vi "Generate DCIR Plots.vi"(8 "error in (no error)":errorcluster, 10 "DCIR Parameters":T1={"Initial SoC (%)"=650.0, "Pulse Mode"=2, "Pulse Current (A)"=1000.0, "Pulse Duration (S)"=500.0} {"Pulse Mode" items=["Discharge"=1, "Charge"=2]; "Initial SoC (%)" min=0.0 max=100.0}, 11 "TDMS Data File":path) -> (0 "error out":errorcluster, 3 "DCIR Nyquist":cluster{dbl[], dbl[]}(graph))   [LabVIEW 2023, in "DCIR_HPPC.lvclass"]
uses:
  HPPC Parameters.ctl
  HPPC Mode.ctl
  <vilib>/Analysis/baseanly.llb/Mean (DBL).vi
  <vilib>/Analysis/2dsp.llb/Real FFT.vi
  DCIR_HPPC.lvclass
  DCIR_HPPC.lvclass/DCIR_HPPC.ctl
  <vilib>/Analysis/NI_AALBase.lvlib
  <vilib>/Analysis/NI_AALPro.lvlib
panel:
  out "dF":dbl
  out "frequency (hz)":dbl
  out "period (seconds)":dbl format="%#_6f"
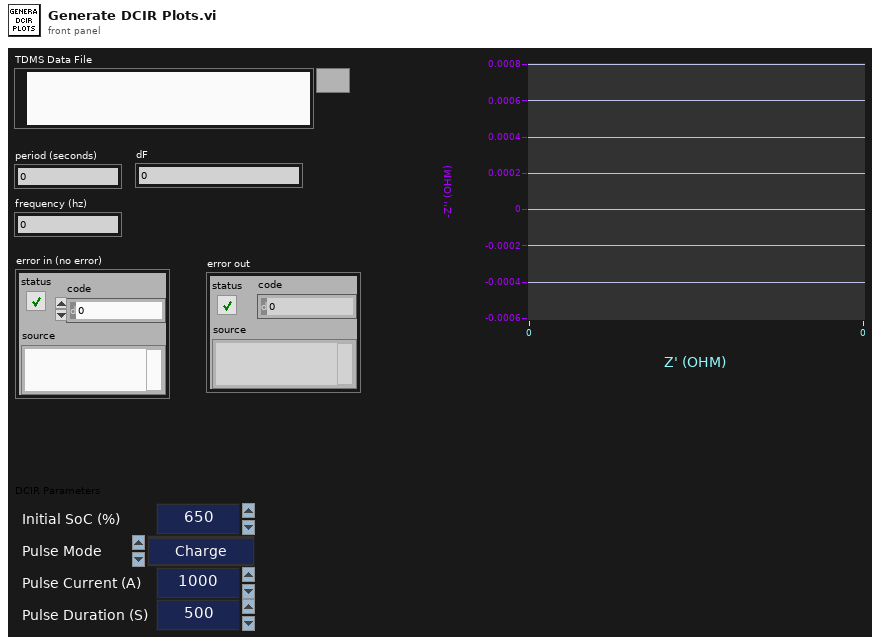
[diagram p1: front panel]
types:
  T1 = typedef "DCIR_HPPC.lvclass/HPPC Parameters.ctl" = cluster{"Initial SoC (%)":dbl, "Pulse Mode":T2, "Pulse Current (A)":dbl, "Pulse Duration (S)":dbl}
  T2 = typedef "DCIR_HPPC.lvclass/HPPC Mode.ctl" = u16
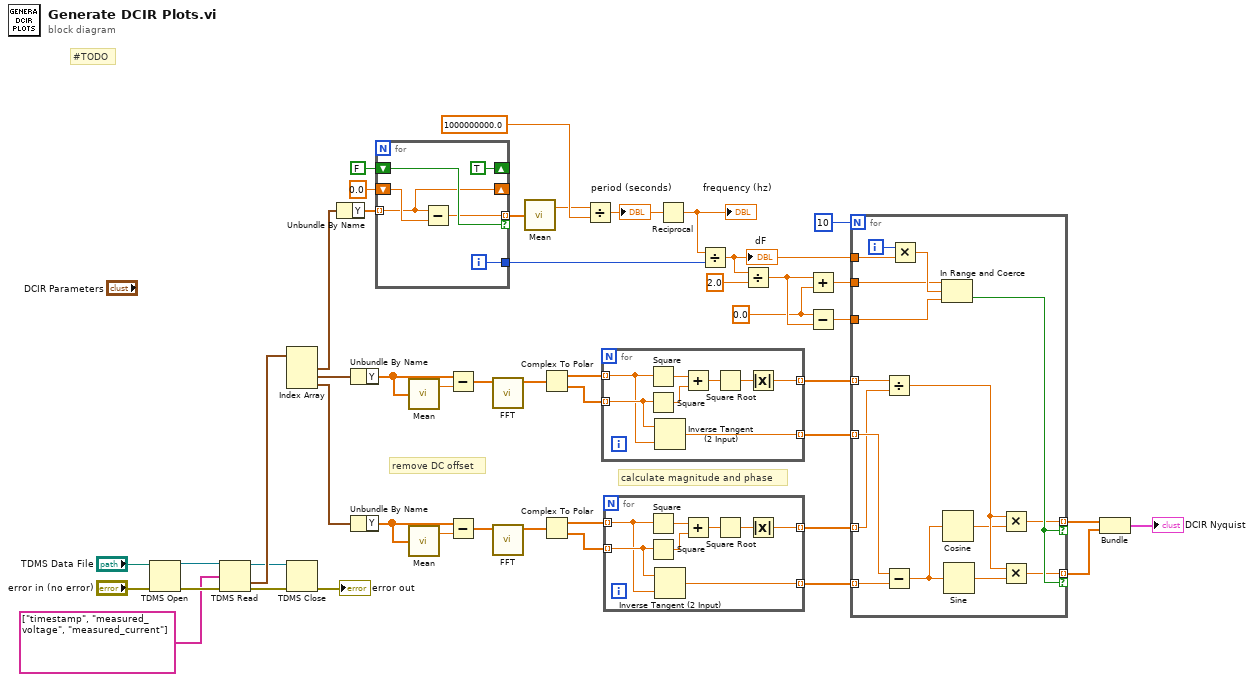
[diagram p0: block diagram]
diagram:
  w2 = 0.0 ("x")
  # "#TODO"
  # "calculate magnitude and phase"
  # "remove DC offset"
  n1 = TDMS Open(8:"error in (no error)", 11:"TDMS Data File") -> (0:w45:errorcluster, 3:w44:refnum<k34>)  [unwired: 5 in]
  n2 = TDMS Read(0:w44, 7:string[] ["timestamp", "measured_voltage", "measured_current"] ("channel name(s) in"), 11:w45) -> (4:w26:refnum<k34>, 10:w42:waveform(dbl)[], 15:w27:errorcluster)  [unwired: 5 in, 3 out]
  n3 = Index Array(array=w42) -> (element #1=w41:waveform(dbl), element #2=w32:waveform(dbl), element #3=w34:waveform(dbl))  [unwired: 3 in]
  n4 = TDMS Close(8:w27, 11:w26) -> (0:→"error out":errorcluster)  [unwired: 1 out]
  n5 = Unbundle By Name(w41) -> ("Y"=w40:dbl[])
  n6 = Unbundle By Name(w32) -> ("Y"=w22:dbl[])
  n7 = Unbundle By Name(w34) -> ("Y"=w18:dbl[])
  n8 = for {
    tunnel: w40 -> [w50] mode=indexing
    tunnel: [w49] -> w38 mode=indexing if=w52
    shift-right: [w50] -> _
    shift-left: 0.0 -> [w51]
    shift-right: [TRUE] -> _
    shift-left: FALSE -> [w52]
    tunnel: [w48] -> w14
    i -> [w48]
    n9 = Subtract(x=w50, y=w51) -> (x-y=w49:dbl)
  }
  n10 = call-poly <vilib>:"Mean.vi"("X"=w22) -> ("mean"=w21:dbl)  [unwired: 1 out]
  n11 = call-poly <vilib>:"Mean.vi"("X"=w18) -> ("mean"=w19:dbl)  [unwired: 1 out]
  n12 = Subtract(x=w22, y=w21) -> (x-y=w20:dbl[])
  n13 = Subtract(x=w18, y=w19) -> (x-y=w17:dbl[])
  n14 = call-poly <vilib>:"FFT.vi"("X"=w20) -> ("FFT {X}"=w13:cdb[])  [unwired: 9 in, 1 out]
  n15 = call-poly <vilib>:"FFT.vi"("X"=w17) -> ("FFT {X}"=w33:cdb[])  [unwired: 9 in, 1 out]
  n16 = call-poly <vilib>:"Mean.vi"("X"=w38) -> ("mean"=w37:dbl)  [unwired: 1 out]
  n17 = Complex To Polar(r * e^(i*theta)=w13) -> (r=w12:dbl[], theta=w28:dbl[])
  n18 = Complex To Polar(r * e^(i*theta)=w33) -> (r=w11:dbl[], theta=w31:dbl[])
  n19 = Divide(x=w37, y=1000000000.0) -> (x/y=w30:dbl)
  "period (seconds)" <- w30
  n20 = for {
    tunnel: w12 -> [w55] mode=indexing
    tunnel: w28 -> [w56] mode=indexing
    tunnel: [w57] -> w16 mode=indexing
    tunnel: [w54] -> w24 mode=indexing
    n21 = Square(x=w55) -> (x^2=w61:dbl)
    n22 = Square(x=w56) -> (x^2=w60:dbl)
    n23 = Inverse Tangent (2 Input)(1:w55, 2:w56) -> (0:w54:dbl)
    n24 = Add(x=w61, y=w60) -> (x+y=w59:dbl)
    n25 = Square Root(x=w59) -> (sqrt(x)=w58:dbl)
    n26 = Absolute Value(x=w58) -> (abs(x)=w57:dbl)
  }
  n27 = for {
    tunnel: w11 -> [w63] mode=indexing
    tunnel: w31 -> [w64] mode=indexing
    tunnel: [w65] -> w29 mode=indexing
    tunnel: [w62] -> w23 mode=indexing
    n28 = Square(x=w63) -> (x^2=w69:dbl)
    n29 = Square(x=w64) -> (x^2=w68:dbl)
    n30 = Inverse Tangent (2 Input)(1:w63, 2:w64) -> (0:w62:dbl)
    n31 = Add(x=w69, y=w68) -> (x+y=w67:dbl)
    n32 = Square Root(x=w67) -> (sqrt(x)=w66:dbl)
    n33 = Absolute Value(x=w66) -> (abs(x)=w65:dbl)
  }
  n34 = Reciprocal(x=w30) -> (1/x=w15:dbl)
  "frequency (hz)" <- w15
  n35 = Divide(x=w15, y=w14) -> (x/y=w10:dbl)
  "dF" <- w10
  n36 = Divide(x=w10, y=2.0) -> (x/y=w8:dbl)
  n37 = Add(x=w8, y=w2) -> (x+y=w6:dbl)
  n38 = Subtract(x=w2, y=w8) -> (x-y=w7:dbl)
  n39 = for {
    N: 10 -> [_]
    tunnel: w16 -> [w80] mode=indexing
    tunnel: w29 -> [w78] mode=indexing
    tunnel: w24 -> [w79] mode=indexing
    tunnel: w23 -> [w81] mode=indexing
    tunnel: [w71] -> w4 mode=indexing if=w72
    tunnel: [w70] -> w3 mode=indexing if=w72
    tunnel: w10 -> [w77]
    tunnel: w7 -> [w73]
    tunnel: w6 -> [w74]
    i -> [w76]
    n40 = Divide(x=w80, y=w78) -> (x/y=w83:dbl)
    n41 = Subtract(x=w79, y=w81) -> (x-y=w85:dbl)
    n42 = Multiply(x=w76, y=w77) -> (x*y=w75:dbl)
    n43 = In Range and Coerce(upper limit=w74, x=w75, lower limit=w73) -> (In Range?=w72:bool)  [unwired: 1 out]
    n44 = Cosine(x=w85) -> (cos(x)=w82:dbl)
    n45 = Sine(x=w85) -> (sin(x)=w84:dbl)
    n46 = Multiply(x=w83, y=w82) -> (x*y=w71:dbl)
    n47 = Multiply(x=w83, y=w84) -> (x*y=w70:dbl)
  }
  n48 = Bundle(w4, w3) -> (→"DCIR Nyquist":cluster{dbl[], dbl[]})  [unwired: 1 in]
